vi "Cal Constants Array to Cluster.vi"(11 "Array":dbl[](array[numeric])) -> (3 "Cluster":T1)   [LabVIEW 2024]
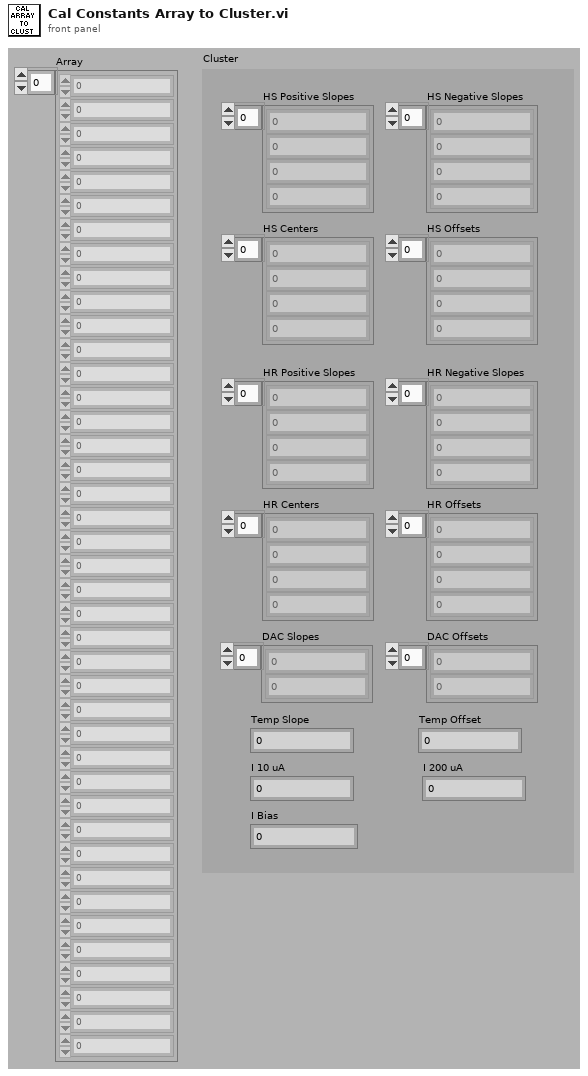
[diagram p1: front panel]
types:
  T1 = cluster{"HS Positive Slopes":dbl[], "HS Negative Slopes":dbl[], "HS Centers":dbl[], "HS Offsets":dbl[], "HR Positive Slopes":dbl[], "HR Negative Slopes":dbl[], "HR Centers":dbl[], "HR Offsets":dbl[], "DAC Slopes":dbl[], "DAC Offsets":dbl[], "Temp Slope":dbl, "Temp Offset":dbl, "I 10 uA":dbl, "I 200 uA":dbl, "I Bias":dbl}
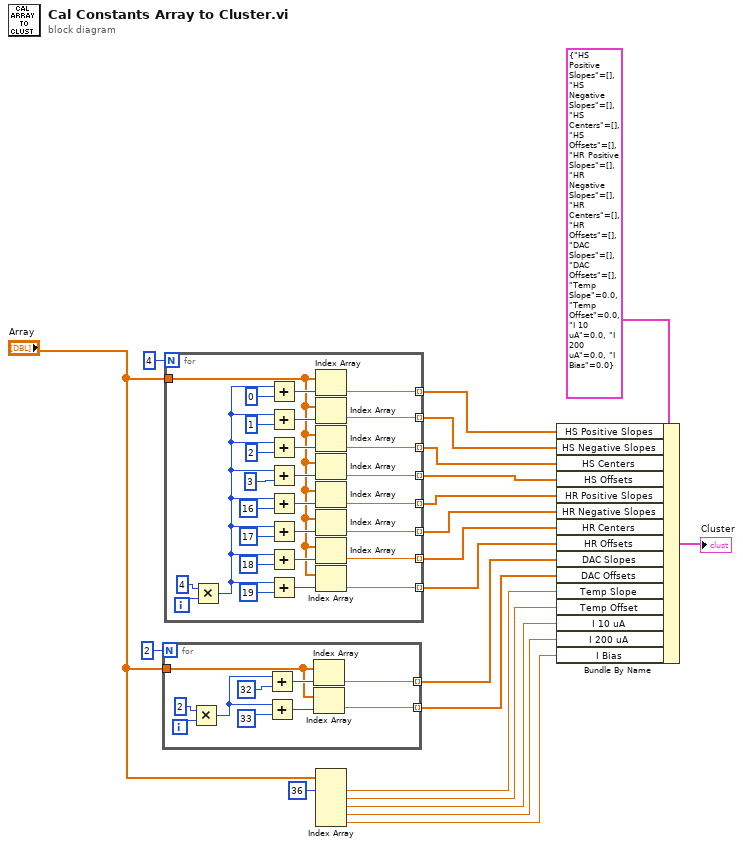
[diagram p0: block diagram]
diagram:
  n1 = for {
    N: 2 -> [_]
    tunnel: "Array" -> [w24]
    tunnel: [w27] -> w7 mode=indexing
    tunnel: [w23] -> w6 mode=indexing
    i -> [w31]
    n2 = Multiply(x=2, y=w31) -> (x*y=w25:i32)
    n3 = Add(x=w25, y=32) -> (x+y=w29:i32)
    n4 = Add(x=w25, y=33) -> (x+y=w26:i32)
    n5 = Index Array(array=w24, index=w29) -> (element=w27:dbl)
    n6 = Index Array(array=w24, index=w26) -> (element=w23:dbl)
  }
  n7 = for {
    N: 4 -> [_]
    tunnel: "Array" -> [w39]
    tunnel: [w55] -> w20 mode=indexing
    tunnel: [w38] -> w19 mode=indexing
    tunnel: [w37] -> w18 mode=indexing
    tunnel: [w36] -> w17 mode=indexing
    tunnel: [w35] -> w16 mode=indexing
    tunnel: [w34] -> w15 mode=indexing
    tunnel: [w33] -> w14 mode=indexing
    tunnel: [w32] -> w13 mode=indexing
    i -> [w59]
    n8 = Multiply(x=4, y=w59) -> (x*y=w40:i32)
    n9 = Add(x=w40, y=0) -> (x+y=w57:i32)
    n10 = Add(x=w40, y=1) -> (x+y=w53:i32)
    n11 = Add(x=w40, y=2) -> (x+y=w52:i32)
    n12 = Add(x=w40, y=3) -> (x+y=w49:i32)
    n13 = Add(x=w40, y=16) -> (x+y=w48:i32)
    n14 = Add(x=w40, y=17) -> (x+y=w45:i32)
    n15 = Add(x=w40, y=18) -> (x+y=w44:i32)
    n16 = Add(x=w40, y=19) -> (x+y=w41:i32)
    n17 = Index Array(array=w39, index=w57) -> (element=w55:dbl)
    n18 = Index Array(array=w39, index=w53) -> (element=w38:dbl)
    n19 = Index Array(array=w39, index=w52) -> (element=w37:dbl)
    n20 = Index Array(array=w39, index=w49) -> (element=w36:dbl)
    n21 = Index Array(array=w39, index=w48) -> (element=w35:dbl)
    n22 = Index Array(array=w39, index=w45) -> (element=w34:dbl)
    n23 = Index Array(array=w39, index=w44) -> (element=w33:dbl)
    n24 = Index Array(array=w39, index=w41) -> (element=w32:dbl)
  }
  n25 = Index Array(array="Array", index #1=36 ("index")) -> (element #1=w5:dbl, element #2=w4:dbl, element #3=w3:dbl, element #4=w2:dbl, element #5=w1:dbl)  [unwired: 4 in]
  n26 = Bundle By Name(cluster=T1 {"HS Positive Slopes"=[], "HS Negative Slopes"=[], "HS Centers"=[], "HS Offsets"=[], "HR Positive Slopes"=[], "HR Negative Slopes"=[], "HR Centers"=[], "HR Offsets"=[], "DAC Slopes"=[], "DAC Offsets"=[], "Temp Slope"=0.0, "Temp Offset"=0.0, "I 10 uA"=0.0, "I 200 uA"=0.0, "I Bias"=0.0} ("Cluster"), "HS Positive Slopes"=w20, "HS Negative Slopes"=w19, "HS Centers"=w18, "HS Offsets"=w17, "HR Positive Slopes"=w16, "HR Negative Slopes"=w15, "HR Centers"=w14, "HR Offsets"=w13, "DAC Slopes"=w7, "DAC Offsets"=w6, "Temp Slope"=w5, "Temp Offset"=w4, "I 10 uA"=w3, "I 200 uA"=w2, "I Bias"=w1) -> (→"Cluster":T1)
